vi "KE2450_Manual_CMDS_Res.vi"() -> ()   [LabVIEW 2017]
uses:
  Instrument Drivers/Keithley 2450/Keithley 2450.lvlib
panel:
  in  "Source Limit Level (0.1)":dbl=0.1
  out "Resistance (ohm)":dbl
  out "error out":errorcluster
  in  "Source Level (1.0)":dbl=1.0
  in  "error in (no error)":errorcluster
  in  "VISA resource name":refnum<visa-resource-name>
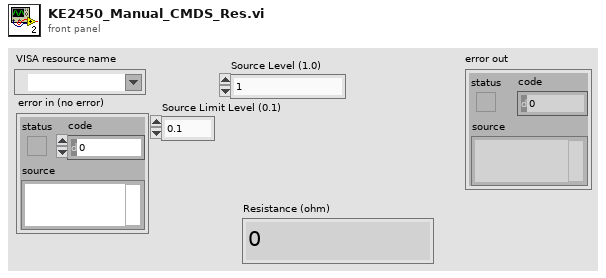
[diagram p1: front panel]
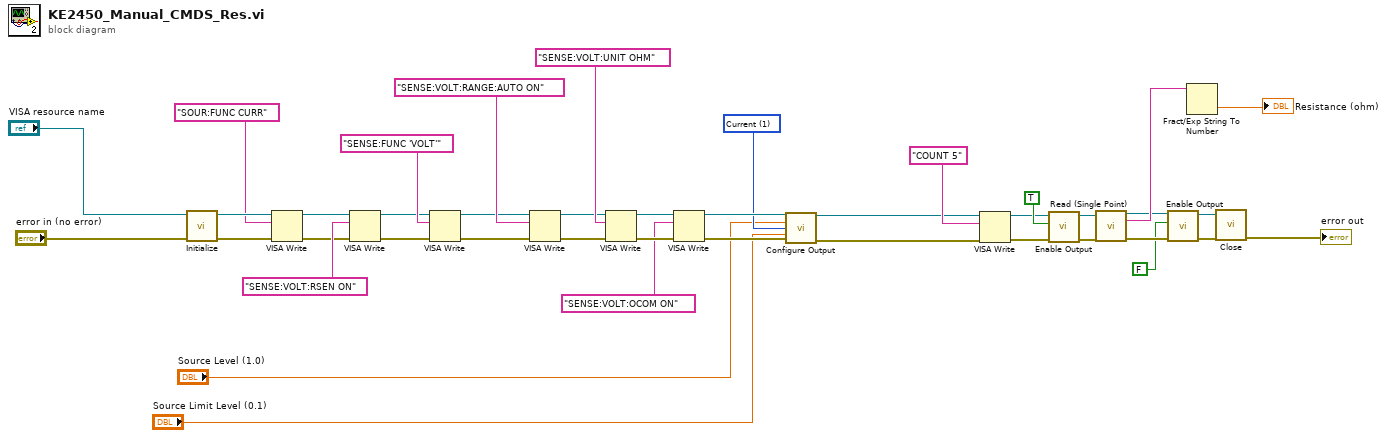
[diagram p0: block diagram]
diagram:
  w21 = u16 1 items=["Voltage", "Current"] ("Source Mode  (0: Voltage)")
  n1 = call "Initialize.vi"("error in (no error)"="error in (no error)", "VISA resource name"="VISA resource name") -> ("error out"=w9:errorcluster, "VISA resource name out"=w8:refnum<visa-resource-name>)  [unwired: 8 in]
  n2 = VISA Write(VISA resource name=w8, write buffer="SOUR:FUNC CURR", error in (no error)=w9) -> (VISA resource name out=w4:refnum<visa-resource-name>, error out=w3:errorcluster)  [unwired: 1 out]
  n3 = VISA Write(VISA resource name=w4, write buffer="SENSE:VOLT:RSEN ON", error in (no error)=w3) -> (VISA resource name out=w1:refnum<visa-resource-name>, error out=w2:errorcluster)  [unwired: 1 out]
  n4 = VISA Write(VISA resource name=w1, write buffer="SENSE:FUNC 'VOLT'", error in (no error)=w2) -> (VISA resource name out=w30:refnum<visa-resource-name>, error out=w31:errorcluster)  [unwired: 1 out]
  n5 = VISA Write(VISA resource name=w30, write buffer="SENSE:VOLT:RANGE:AUTO ON", error in (no error)=w31) -> (VISA resource name out=w28:refnum<visa-resource-name>, error out=w27:errorcluster)  [unwired: 1 out]
  n6 = VISA Write(VISA resource name=w28, write buffer="SENSE:VOLT:UNIT OHM", error in (no error)=w27) -> (VISA resource name out=w26:refnum<visa-resource-name>, error out=w25:errorcluster)  [unwired: 1 out]
  n7 = VISA Write(VISA resource name=w26, write buffer="SENSE:VOLT:OCOM ON", error in (no error)=w25) -> (VISA resource name out=w22:refnum<visa-resource-name>, error out=w23:errorcluster)  [unwired: 1 out]
  n8 = call "Configure Output.vi"("VISA resource name"=w22, "Source Level (0)"="Source Level (1.0)", "Source Mode  (0: Voltage)"=w21, "Source Limit Level (0.1)"="Source Limit Level (0.1)", "error in (no error)"=w23) -> ("VISA resource name out"=w5:refnum<visa-resource-name>, "error out"=w6:errorcluster)  [unwired: 9 in]
  n9 = VISA Write(VISA resource name=w5, write buffer="COUNT 5", error in (no error)=w6) -> (VISA resource name out=w17:refnum<visa-resource-name>, error out=w16:errorcluster)  [unwired: 1 out]
  n10 = call "Enable Output.vi"("error in (no error)"=w16, "Enable Output (T: Enable)"=TRUE, "VISA resource name"=w17) -> ("error out"=w37:errorcluster, "VISA resource name out"=w36:refnum<visa-resource-name>)  [unwired: 7 in]
  n11 = call "Read (Single Point).vi"("VISA resource name"=w36, "error in (no error)"=w37) -> ("VISA resource name out"=w12:refnum<visa-resource-name>, "Data out"=w34:string, "error out"=w13:errorcluster)  [unwired: 11 in]
  n12 = call "Enable Output.vi"("error in (no error)"=w13, "Enable Output (T: Enable)"=FALSE, "VISA resource name"=w12) -> ("error out"=w15:errorcluster, "VISA resource name out"=w14:refnum<visa-resource-name>)  [unwired: 7 in]
  n13 = Fract/Exp String To Number(string=w34) -> (number=→"Resistance (ohm)":dbl)  [unwired: 3 in, 1 out]
  n14 = call "Close.vi"("error in (no error)"=w15, "VISA resource name"=w14) -> ("error out"=→"error out":errorcluster)  [unwired: 9 in]
